vi "_CalDialog.vi"(9 "ChangeFreq":bool, 10 "Частота, Гц":dbl=150000.0 min=1000.0 max=1000000.0) -> (1 "ArrayFreq":dbl[](array[numeric]), 3 "Cancelled?":bool)   [LabVIEW 2017]
doc: "Use this template to create a dialog box with event handling."
uses:
  st_str Global.vi
  <vilib>/Utility/file.llb/Read Delimited Spreadsheet (string).vi
  <vilib>/Utility/file.llb/Write Delimited Spreadsheet (string).vi
panel:
  out "appended path":path
  in  "Interpolation factor (n)":i32 min=0 max=10 step=1
  in  "Table":string[][](table)=[["", "50000", "100000", "200000"], ["100", "0", "0", "0"], ["75.3", "-11.3", "-21.7", "-46.55"], ["55.3", "-19.9", "-30.2", "-69.65"], ["35.3", "-30", "-47.2", "-109.2"], ["14.7", "-35.5", "-55.6", "-127.5"], ["10", "-38.8", "-61.8", "-138.6"]]
  in  "Load":bool
  in  "Save":bool
  out "XY_deap_phase":cluster{"Data":dbl[], "Data":dbl[]}[](graph) caption="XY График"
  in  "Cancel":bool
  in  "OK":bool
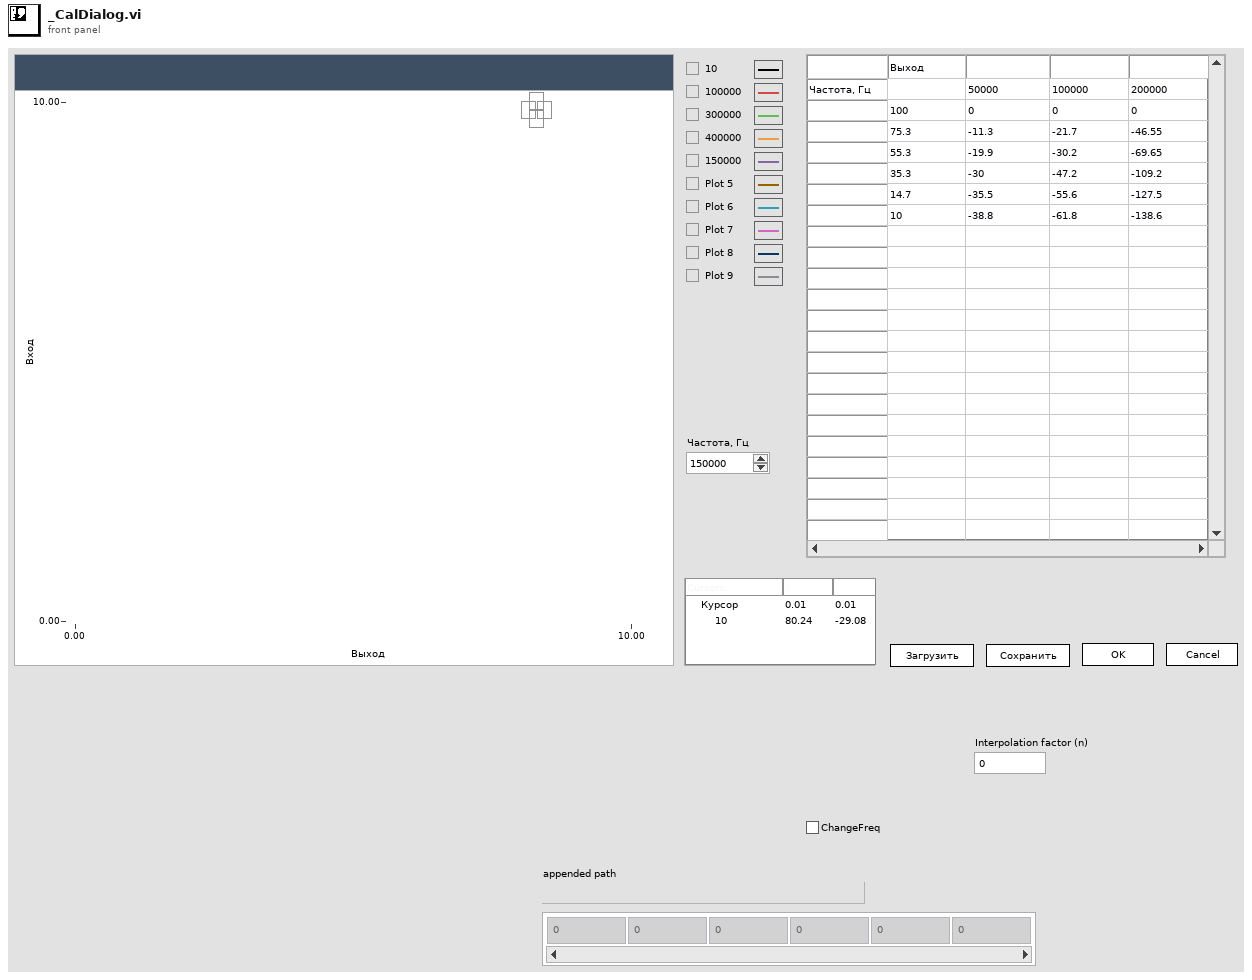
[diagram p1: front panel]
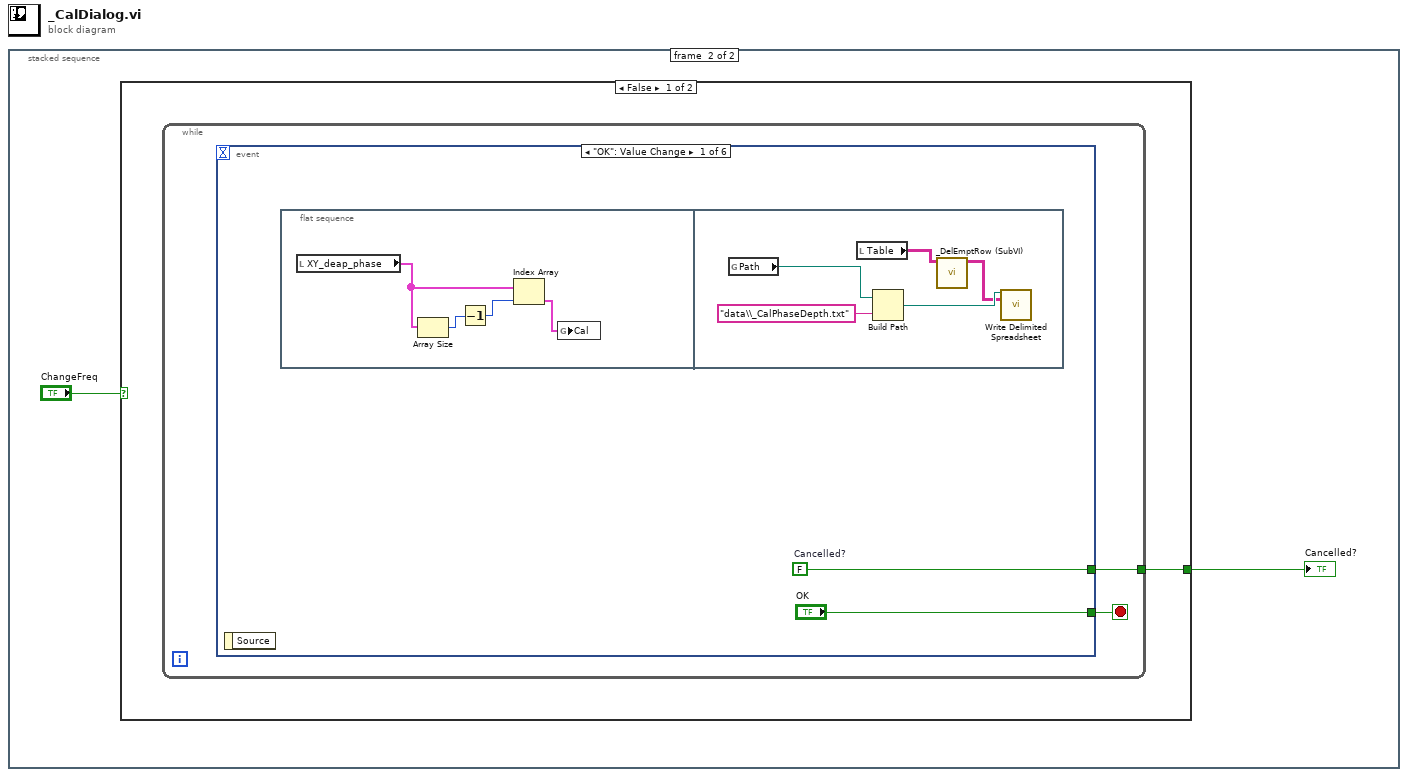
[diagram p0: block diagram]
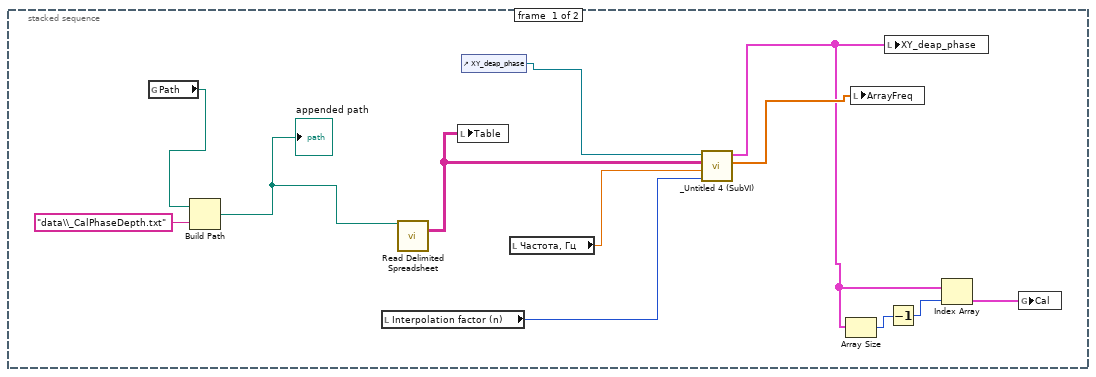
[diagram p2: hidden frame]
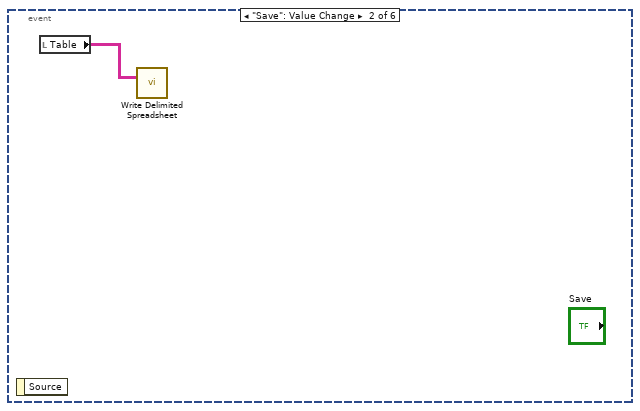
[diagram p3: hidden frame]
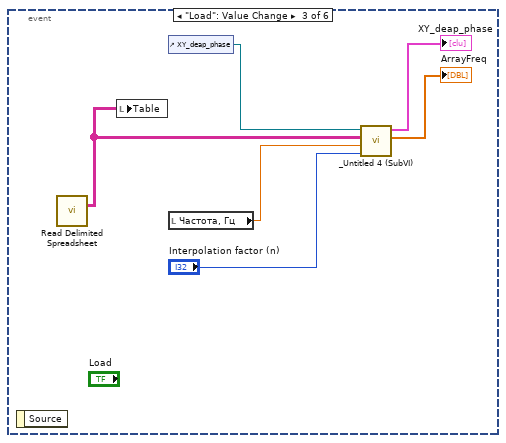
[diagram p4: hidden frame]
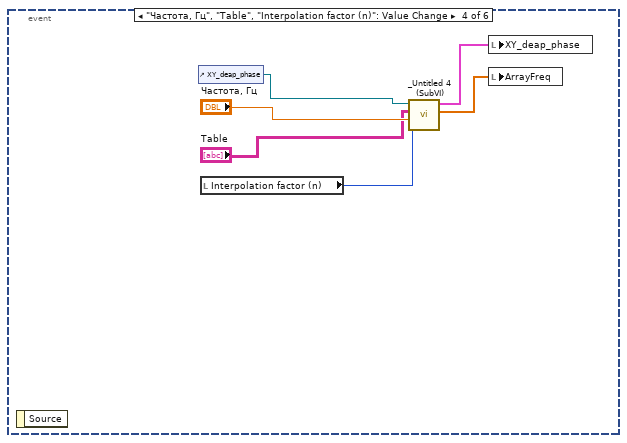
[diagram p5: hidden frame]
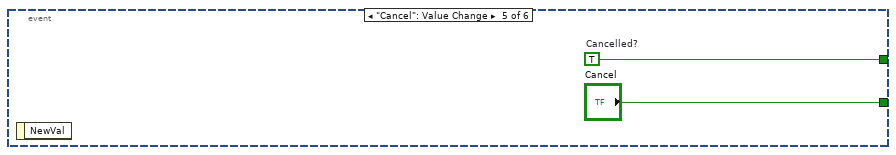
[diagram p6: hidden frame]
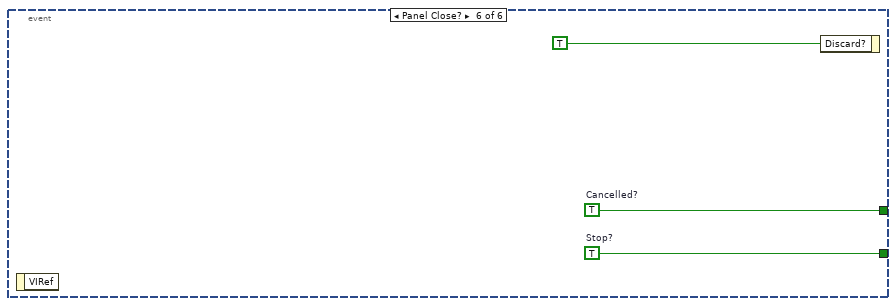
[diagram p7: hidden frame]
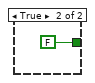
[diagram p8: hidden frame]
diagram:
  n1 = stacked-sequence {
    frame #0 {
      n2 = global read "st_str Global.vi" "Path"() -> (w1:path)
      n3 = Build Path(base path=w1, name or relative path="data\\_CalPhaseDepth.txt") -> (appended path=w6:path)
      "appended path" <- w6
      n4 = local read "Interpolation factor (n)"() -> (w10:i32)
      n5 = call-poly <vilib>:"Read Delimited Spreadsheet.vi"("file path (dialog if empty)"=w6) -> ("all rows"=w8:string[][])  [unwired: 9 in, 5 out]
      n6 = local write "Table"(w8) -> ()
      n7 = control-ref of="XY_deap_phase"() -> (w11:refnum<vi>)
      n8 = local read "Частота, Гц"() -> (w9:dbl)
      n9 = call "_Untitled 4 (SubVI).vi"("Interpolation factor (n)"=w10, "Частота, Гц"=w9, "all rows"=w8, "XYGraph in"=w11) -> ("ArrayFreqOut"=w12:dbl[], "ArrayOut"=w2:cluster{dbl[], dbl[]}[])  [unwired: 6 in]
      n10 = Array Size(array=w2) -> (size(s)=w5:i32)
      n11 = local write "ArrayFreq"(w12) -> ()
      n12 = local write "XY_deap_phase"(w2) -> ()
      n13 = Decrement(x=w5) -> (x-1=w4:i32)
      n14 = Index Array(array=w2, index=w4) -> (element=w3:cluster{dbl[], dbl[]})
      n15 = global write "st_str Global.vi" "Cal"(w3) -> ()
    }
    frame #1 {
      n16 = case shown="False" "ChangeFreq" {
        tunnel: [w15 FALSE ("Cancelled?")] -> w14
        frame False {
          n17 = while {
            tunnel: [w16] -> w15
            stop <- w17 stop-if-true
            n18 = event shown="[0] \"OK\": Value Change" {
              selector: _ -> [_ _ _ _ _ _]
              dyn-events: _ -> [_ _ _ _ _ _]
              timeout: _ -> [_ _ _ _ _ _]
              tunnel: ["OK" _ _ _ "Cancel" w45] -> w17
              tunnel: [w19 _ _ _ w43 w44] -> w16
              event "OK": Value Change {
                w19 = FALSE  # Cancelled?
                n19 = event-data() -> ()  [unwired: 1 in, 1 out]
                n20 = flat-sequence {
                  frame #0 {
                    n21 = local read "XY_deap_phase"() -> (w23:cluster{"Data":dbl[], "Data":dbl[]}[])
                    n22 = Array Size(array=w23) -> (size(s)=w22:i32)
                    n23 = Decrement(x=w22) -> (x-1=w21:i32)
                    n24 = Index Array(array=w23, index=w21) -> (element=w20:cluster{"Data":dbl[], "Data":dbl[]})
                    n25 = global write "st_str Global.vi" "Cal"(w20) -> ()
                  }
                  frame #1 {
                    n26 = global read "st_str Global.vi" "Path"() -> (w27:path)
                    n27 = local read "Table"() -> (w25:string[][])
                    n28 = Build Path(base path=w27, name or relative path="data\\_CalPhaseDepth.txt") -> (appended path=w28:path)
                    n29 = call "_DelEmptRow (SubVI).vi"("all rows in"=w25) -> ("all rows out"=w24:string[][])  [unwired: 10 in]
                    n30 = call-poly <vilib>:"Write Delimited Spreadsheet.vi"("file path (dialog if empty)"=w28, "2D data"=w24) -> ()  [unwired: 12 in, 2 out]
                  }
                }
              }
              event "Save": Value Change {
                n31 = event-data() -> ()  [unwired: 1 in, 1 out]
                n32 = local read "Table"() -> (w29:string[][])
                n33 = call-poly <vilib>:"Write Delimited Spreadsheet.vi"("2D data"=w29) -> ()  [unwired: 13 in, 2 out]
              }
              event "Load": Value Change {
                n34 = event-data() -> ()  [unwired: 1 in, 1 out]
                n35 = call-poly <vilib>:"Read Delimited Spreadsheet.vi"() -> ("all rows"=w30:string[][])  [unwired: 10 in, 5 out]
                n36 = local write "Table"(w30) -> ()
                n37 = control-ref of="XY_deap_phase"() -> (w34:refnum<vi>)
                n38 = local read "Частота, Гц"() -> (w35:dbl)
                n39 = call "_Untitled 4 (SubVI).vi"("Interpolation factor (n)"="Interpolation factor (n)", "Частота, Гц"=w35, "all rows"=w30, "XYGraph in"=w34) -> ("ArrayFreqOut"=→"ArrayFreq":dbl[], "ArrayOut"=→"XY_deap_phase":cluster{dbl[], dbl[]}[])  [unwired: 6 in]
              }
              event "Частота, Гц", "Table", "Interpolation factor (n)": Value Change {
                n40 = event-data() -> ()  [unwired: 1 in, 1 out]
                n41 = control-ref of="XY_deap_phase"() -> (w41:refnum<vi>)
                n42 = local read "Interpolation factor (n)"() -> (w37:i32)
                n43 = call "_Untitled 4 (SubVI).vi"("Interpolation factor (n)"=w37, "Частота, Гц"="Частота, Гц", "all rows"="Table", "XYGraph in"=w41) -> ("ArrayFreqOut"=w38:dbl[], "ArrayOut"=w39:cluster{dbl[], dbl[]}[])  [unwired: 6 in]
                n44 = local write "XY_deap_phase"(w39) -> ()
                n45 = local write "ArrayFreq"(w38) -> ()
              }
              event "Cancel": Value Change {
                w43 = TRUE  # Cancelled?
                n46 = event-data() -> ()  [unwired: 1 in, 1 out]
              }
              event Panel Close? {
                w44 = TRUE  # Cancelled?
                w45 = TRUE  # Stop?
                n47 = event-data() -> ()  [unwired: 1 in, 1 out]
                n48 = event-data("Discard?"=TRUE) -> ()  [unwired: 1 in, 1 out]
              }
            }
          }
        }
        frame True {
        }
      }
      "Cancelled?" <- w14
    }
  }
